vi "MainFGV.vi"(7 "FGV_mods":T1, 8 "Error In":errorcluster, 11 "DataIn":variant) -> (0 "Error Out":errorcluster, 3 "DataOut":variant)   [LabVIEW 2016]
uses:
  CurrentMeter/CM_SerialNumber.ctl
  CurrentMeter/CM_data.ctl
  StrainGauge/SG_data.ctl
  MainFGV_data.ctl
  <vilib>/Utility/config.llb/NI_LVConfig.lvlib
  MainFGV_mods.ctl
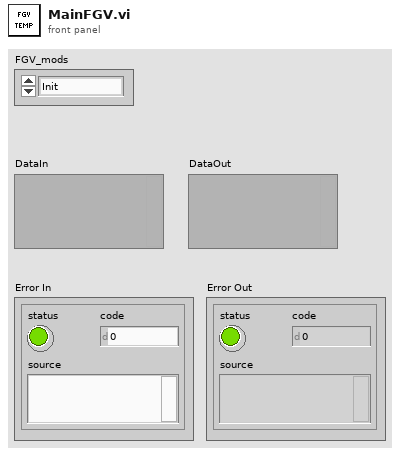
[diagram p1: front panel]
types:
  T1 = typedef "MainFGV_mods.ctl" = enum16{"Init", "Config", "CreateTask", "Register", "Start", "Record", "End"}
  T2 = cluster{"simulation":bool, "TesrtDir":path, "TestName":string}
  T3 = typedef "MainFGV_data.ctl" = cluster{"TestDir":path, "TestName":string, "CM_data":T4[], "SG_data":T6[], "Simulation":bool}
  T4 = typedef "CM_data.ctl" = cluster{"Serial":T5, "Coordenada X":dbl, "Coordenada Y":dbl, "ID":string, "active":bool}
  T5 = typedef "CM_SerialNumber.ctl" = enum16{"274124", "274125", "274126", "274127", "274128"}
  T6 = typedef "SG_data.ctl" = cluster{"ID":string, "Sensibilidade":dbl, "Descrição":string, "active":bool}
  T7 = typedef "NI_LVConfig.lvlib/Config Data RefNum.ctl" = refnum<k1>
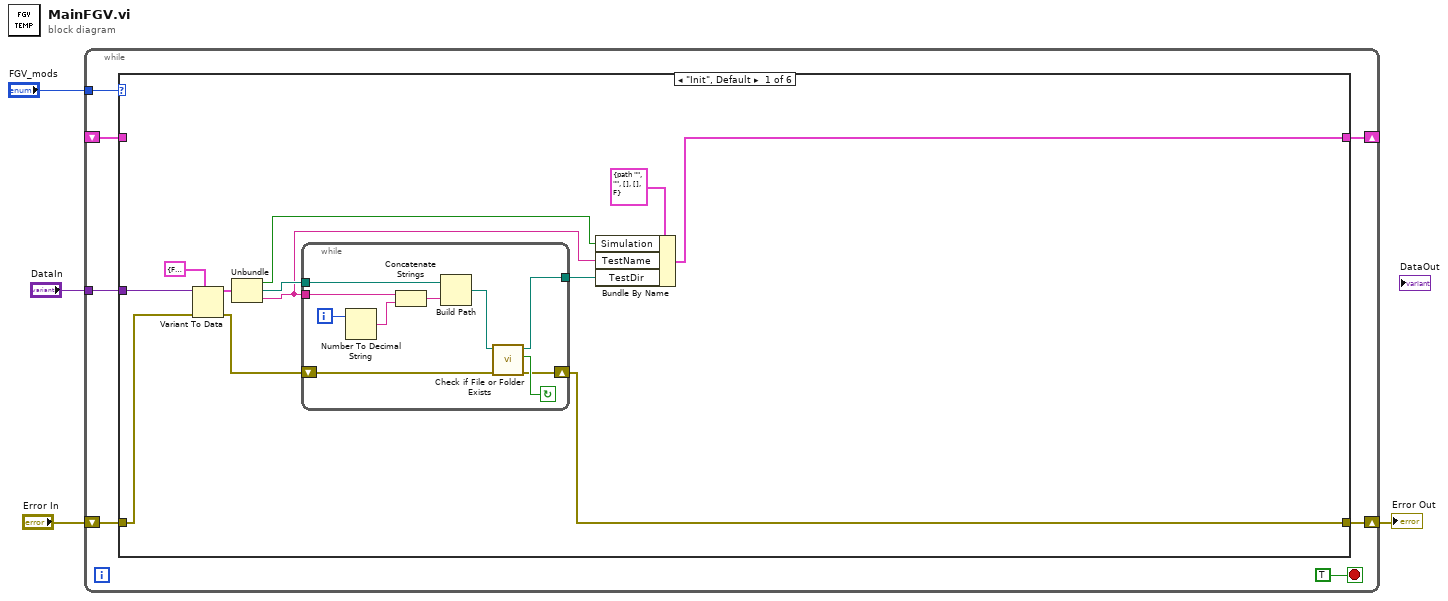
[diagram p0: block diagram]
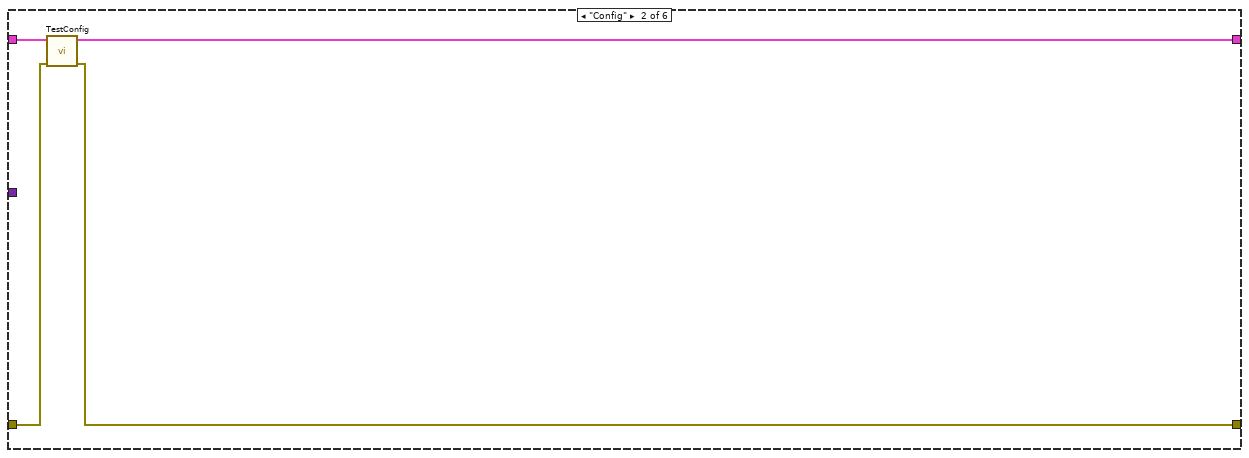
[diagram p2: hidden frame]
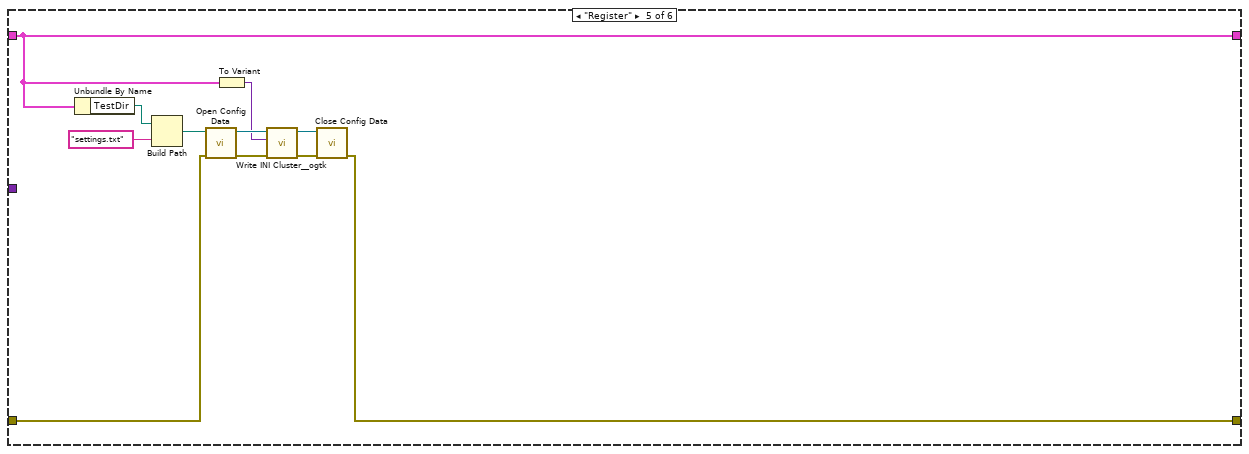
[diagram p5: hidden frame]
diagram:
  n1 = while {
    tunnel: "DataIn" -> [w10]
    tunnel: "FGV_mods" -> [w9]
    shift-right: [w8] -> _
    shift-left: _ -> [w7]
    shift-right: [w5] -> w1
    shift-left: "Error In" -> [w6]
    stop <- TRUE stop-if-true
    n2 = case shown="\"Init\", Default" w9 {
      tunnel: w10 -> [w23 _ _ _ _ _]
      tunnel: [w19 w35 w39 _ w40 _] -> w8
      tunnel: w7 -> [_ w37 w39 _ w40 _]
      tunnel: w6 -> [w22 w36 w38 _ w47 _]
      tunnel: [w16 w34 w38 _ w41 _] -> w5
      frame "Init", Default {
        n3 = Variant To Data(error in=w22, type=T2 {"simulation"=FALSE, "TesrtDir"=path "", "TestName"=""} ("output cluster"), Variant=w23) -> (data=w20:T2, error out=w18:errorcluster)
        n4 = Unbundle(w20) -> ("simulation"=w12:bool, "TesrtDir"=w14:path, "TestName"=w13:string)
        n5 = while {
          tunnel: w13 -> [w31]
          tunnel: w14 -> [w29]
          shift-right: [w25] -> w16
          shift-left: w18 -> [w27]
          tunnel: [w24] -> w17
          i -> [w33]
          stop <- w26 continue-if-true
          n6 = Number To Decimal String(number=w33) -> (decimal integer string=w32:string)  [unwired: 1 in]
          n7 = Concatenate Strings(w31, w32) -> (w30:string)
          n8 = Build Path(base path=w29, name or relative path=w30) -> (appended path=w28:path)
          n9 = call <vilib>:"Check if File or Folder Exists.vi"("error in (no error)"=w27, "path"=w28) -> ("error out"=w25:errorcluster, "file or folder exists?"=w26:bool, "dup path"=w24:path)  [unwired: 7 in]
        }
        n10 = Bundle By Name(cluster=T3 {"TestDir"=path "", "TestName"="", "CM_data"=[], "SG_data"=[], "Simulation"=FALSE} ("MainFGV_data"), "Simulation"=w12, "TestName"=w13, "TestDir"=w17) -> (w19:T3)
      }
      frame "Config" {
        n11 = call "TestConfig.vi"("error in"=w36, "MainFGV_data"=w37) -> ("error out"=w34:errorcluster, "MainFGV_data out"=w35:T3)  [unwired: 8 in]
      }
      frame "End" {
      }
      frame "CreateTask" {
      }
      frame "Register" {
        n12 = Unbundle By Name(w40) -> ("TestDir"=w50:path)
        n13 = Build Path(base path=w50, name or relative path="settings.txt") -> (appended path=w48:path)
        n14 = call <vilib>:"Open Config Data.vi"("error in (no error)"=w47, "configuration file path"=w48) -> ("error out"=w44:errorcluster, "refnum"=w46:T7)  [unwired: 7 in, 1 out]
        n15 = To Variant(anything=w40) -> (Variant=w45:variant)
        n16 = call <userlib>:"Write INI Cluster__ogtk.vi"("error in (no error)"=w44, "INI Fomatted Cluster"=w45, "refnum"=w46) -> ("error out"=w43:errorcluster, "dup refnum"=w42:T7)  [unwired: 7 in]
        n17 = call <vilib>:"Close Config Data.vi"("error in (no error)"=w43, "refnum"=w42) -> ("error out"=w41:errorcluster)  [unwired: 8 in, 1 out]
      }
      frame "Record" {
      }
    }
  }
  "Error Out" <- w1
